vi "cRIO Benchmarking PC Main.vi"() -> ()   [LabVIEW 2013]
doc: "This application launches and executes the Tag Bus Data framework configuration for the specified target alias. This is a simple example of the framework API functions, but may also be a suitable starting point for a Host UI or Thick Client that is running a local version of the framework."
uses:
  <vilib>/NI/Module Execution Interface/Engine Runtime/Execution States.ctl
  <vilib>/NI/Module Execution Interface/Engine Runtime/Fault.ctl
  <vilib>/NI/Tag Bus Module Framework/runtime/error classification.ctl
  <vilib>/NI/Module Execution Interface/Engine Runtime/Engine Runtime Interface.lvclass
  <vilib>/NI/DCAF/Tag Editor Core/Framework Configuration Classes/target runtime/PL_Target Runtime.lvclass
  <vilib>/NI/Tag Bus Module Framework/runtime/TBM module execution interface.lvclass
panel:
  in  "File Name in Root Directory":string="Integration Testing Configuration.pcfg"
  in  "target alias":string="cRIO Benchmarking UI"
  out "engine status":T4(array[cluster])
  in  "stop":bool
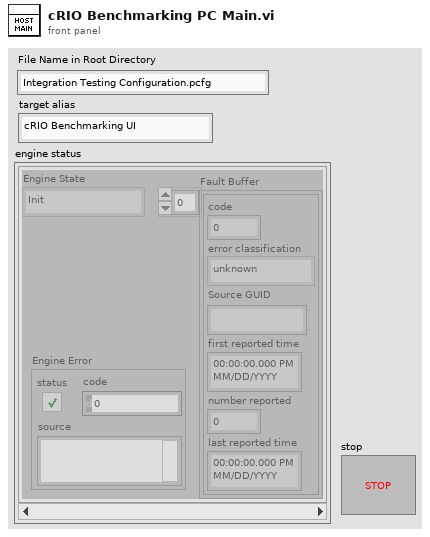
[diagram p1: front panel]
types:
  T1 = typedef "Engine Runtime Interface.lvclass/Execution States.ctl" = enum16{"Init", "Pre-Operational", "Safe-Operational", "Operational", "Stopped"}
  T2 = typedef "Engine Runtime Interface.lvclass/Fault.ctl" = cluster{"code":i32, "error classification":T3, "Source GUID":string, "first reported time":timestamp, "number reported":u32, "last reported time":timestamp}
  T3 = typedef "TBM module execution interface.lvclass/error classification.ctl" = enum16{"unknown", "none", "trivial", "recoverable", "critical"}
  T4 = cluster{"Engine State":T1, "Fault Buffer":T2[], "Engine Error":errorcluster}[]
  T5 = cluster{"Engine State":T1, "faults":T2[], "Engine Error":errorcluster}
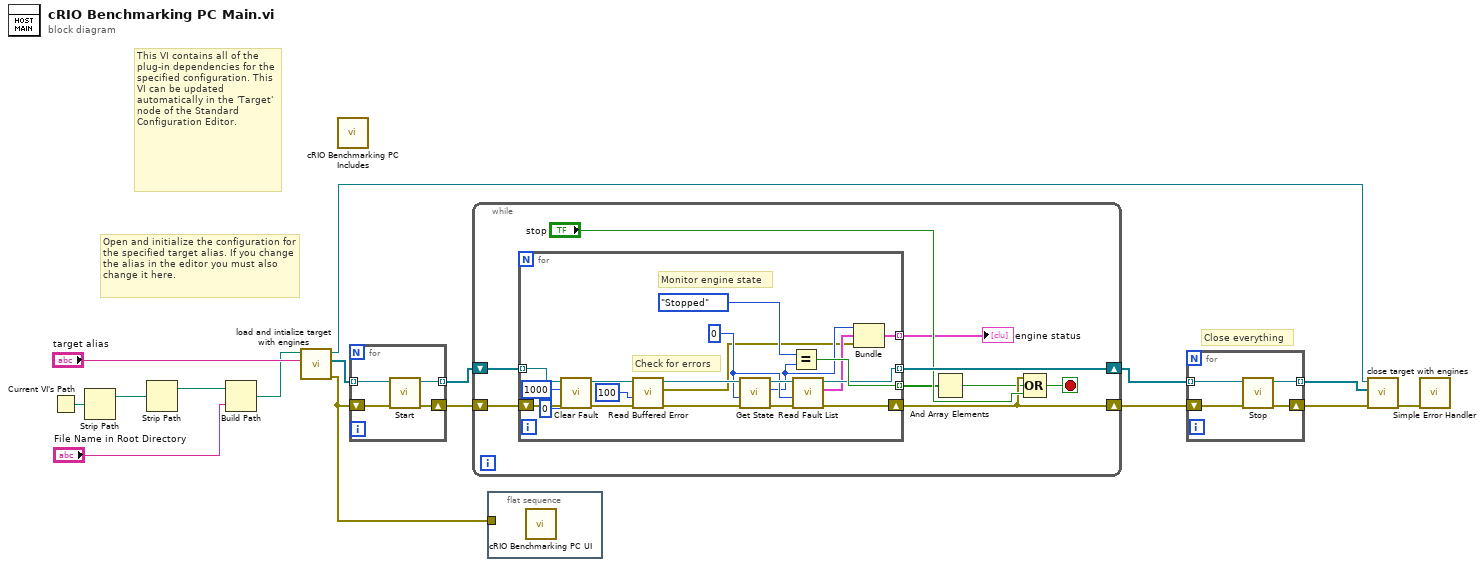
[diagram p0: block diagram]
diagram:
  # "Open and initialize the configuration for the specified target alias. If you change the alias in the editor you must also change it here."
  # "Close everything"
  # "This VI contains all of the plug-in dependencies for the specified configuration. This VI can be updated automatically in the 'Target' node of the Standard Configuration Editor."
  n1 = Current VI's Path() -> (path=w6:path)
  n2 = Strip Path(path=w6) -> (stripped path=w4:path)  [unwired: 1 out]
  n3 = Strip Path(path=w4) -> (stripped path=w3:path)  [unwired: 1 out]
  n4 = Build Path(base path=w3, name or relative path="File Name in Root Directory") -> (appended path=w1:path)
  n5 = call <vilib>:"load and intialize target with engines.vi"("target alias"="target alias", "file path"=w1) -> ("error out"=w8:errorcluster, "engine runtime interfaces"=w13:refnum<class "Engine Runtime Interface.lvclass">[], "target runtime"=w10:refnum<class "PL_Target Runtime.lvclass">)  [unwired: 7 in]
  n6 = call "cRIO Benchmarking PC Includes.vi"() -> ()  [unwired: 12 in]
  n7 = for {
    tunnel: [w20] -> w16 mode=indexing
    tunnel: w13 -> [w17] mode=indexing
    shift-right: [w19] -> w7
    shift-left: w8 -> [w18]
    n8 = call-dynamic "Start.vi"("error in"=w18, "Engine Runtime Interface in"=w17) -> ("error out"=w19:errorcluster, "Engine Runtime Interface out"=w20:refnum<class "Engine Runtime Interface.lvclass">)  [unwired: 8 in]
  }
  n9 = while {
    shift-right: [w27] -> w15
    shift-left: w16 -> [w29]
    shift-right: [w24] -> w14
    shift-left: w7 -> [w28]
    stop <- w25 stop-if-true
    n10 = for {
      tunnel: w29 -> [w33] mode=indexing
      tunnel: [w42] -> w27 mode=indexing
      tunnel: [w46] -> w22 mode=indexing
      shift-right: [w41] -> w24
      shift-left: w28 -> [w35]
      tunnel: [w36] -> w23 mode=indexing
      w40 = 0 ("timeout (-1)")
      # "Monitor engine state"
      # "Check for errors"
      n11 = call-dynamic "Clear Fault.vi"("error in"=w35, "timeout (-1)"=0, "code (0=clear all)"=1000, "Engine Runtime Interface in"=w33) -> ("error out"=w34:errorcluster, "Engine Runtime Interface out"=w32:refnum<class "Engine Runtime Interface.lvclass">)  [unwired: 6 in]
      n12 = call-dynamic "Read Buffered Error.vi"("error in"=w34, "timeout in ms (0)"=100, "Engine Runtime Interface in"=w32) -> ("error out"=w48:errorcluster, "Engine Error"=w37:errorcluster, "Engine Runtime Interface out"=w49:refnum<class "Engine Runtime Interface.lvclass">)  [unwired: 6 in]
      n13 = call-dynamic "Get State.vi"("error in"=w48, "timeout (-1)"=w40, "Engine Runtime Interface in"=w49) -> ("error out"=w44:errorcluster, "Engine State"=w39:T1, "Engine Runtime Interface out"=w43:refnum<class "Engine Runtime Interface.lvclass">)  [unwired: 6 in]
      n14 = Equal?(x=Execution_States."Stopped" ("Engine State"), y=w39) -> (x = y?=w46:bool)
      n15 = call-dynamic "Read Fault List.vi"("error in"=w44, "timeout (-1)"=w40, "Engine Runtime Interface in"=w43) -> ("error out"=w41:errorcluster, "faults"=w38:T2[], "Engine Runtime Interface out"=w42:refnum<class "Engine Runtime Interface.lvclass">)  [unwired: 6 in]
      n16 = Bundle("Engine State"=w39, "faults"=w38, "Engine Error"=w37) -> (w36:T5)  [unwired: 1 in]
    }
    "engine status" <- w23
    n17 = And Array Elements(Boolean array=w22) -> (logical AND=w21:bool)
    n18 = Compound Arithmetic op=OR(w24, w21, "stop") -> (w25:bool)
  }
  n19 = flat-sequence {
    tunnel: w8 -> [_]
    frame #0 {
      n20 = call "cRIO Benchmarking PC UI.vi"() -> ()  [unwired: 12 in]
    }
  }
  n21 = for {
    tunnel: w15 -> [w53] mode=indexing
    shift-right: [w50] -> w9
    shift-left: w14 -> [w52]
    tunnel: [w51] -> w11 mode=indexing
    n22 = call-dynamic "Stop.vi"("error in"=w52, "Engine Runtime Interface in"=w53) -> ("error out"=w50:errorcluster, "Engine Runtime Interface out"=w51:refnum<class "Engine Runtime Interface.lvclass">)  [unwired: 8 in]
  }
  n23 = call <vilib>:"close target with engines.vi"("error in"=w9, "Engine Runtime Interfaces"=w11, "Target Runtime"=w10) -> ("error out"=w5:errorcluster)  [unwired: 8 in]
  n24 = call <vilib>:"Simple Error Handler.vi"("error in (no error)"=w5) -> ()  [unwired: 4 in, 5 out]
